vi "calculate_resistance.vi"(0 "Bare Resistance (MOhm)":dbl, 1 "Live Resistance":dbl, 2 "Solution Conductance \nS/m":dbl, 3 "Sealed Resistance (MOhm)":dbl, 5 "Membrane Thickness (nm)":dbl, 6 "Override":bool, 7 "Desired Pore Size (nm)":dbl) -> (4 "Boolean":bool, 10 "Capillary Diameter (nm)":dbl, 16 "Target Golovochenko  (MOhm)":dbl)   [LabVIEW 2016]
panel:
  out "Alpha":dbl
  out "Beta":dbl
  out "Membrane Thickness (m)":dbl
  out "Target Pore Diameter (m)":dbl
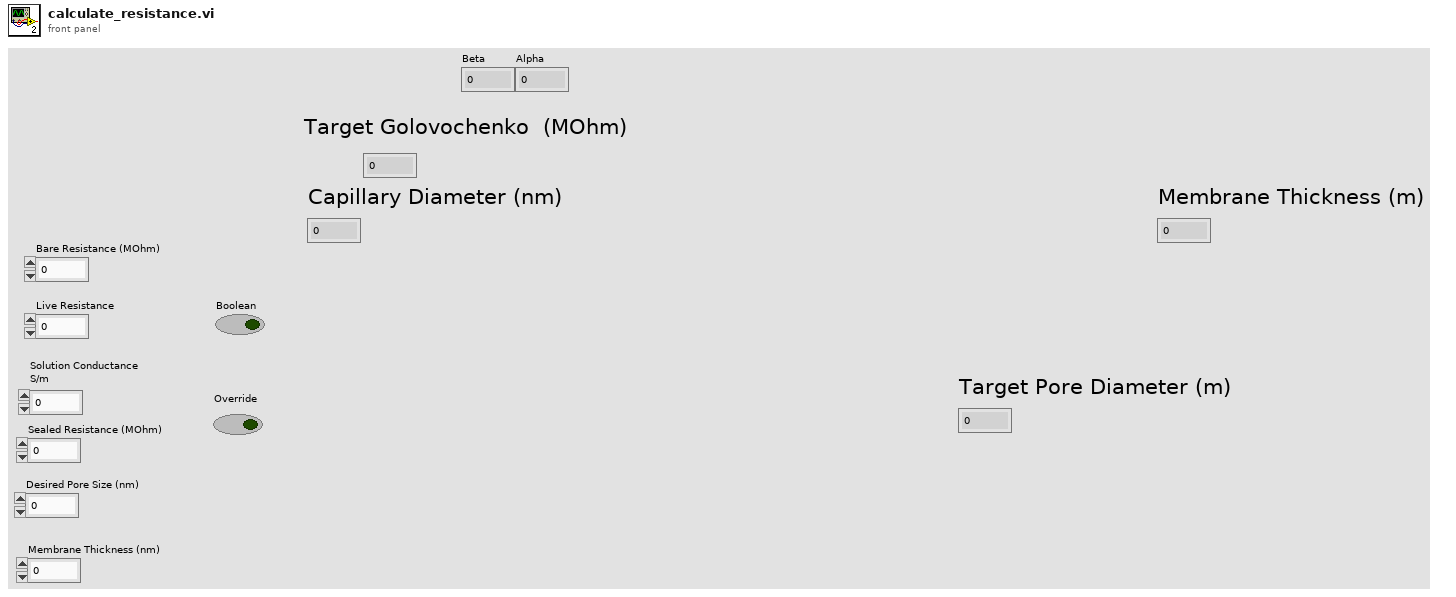
[diagram p1: front panel]
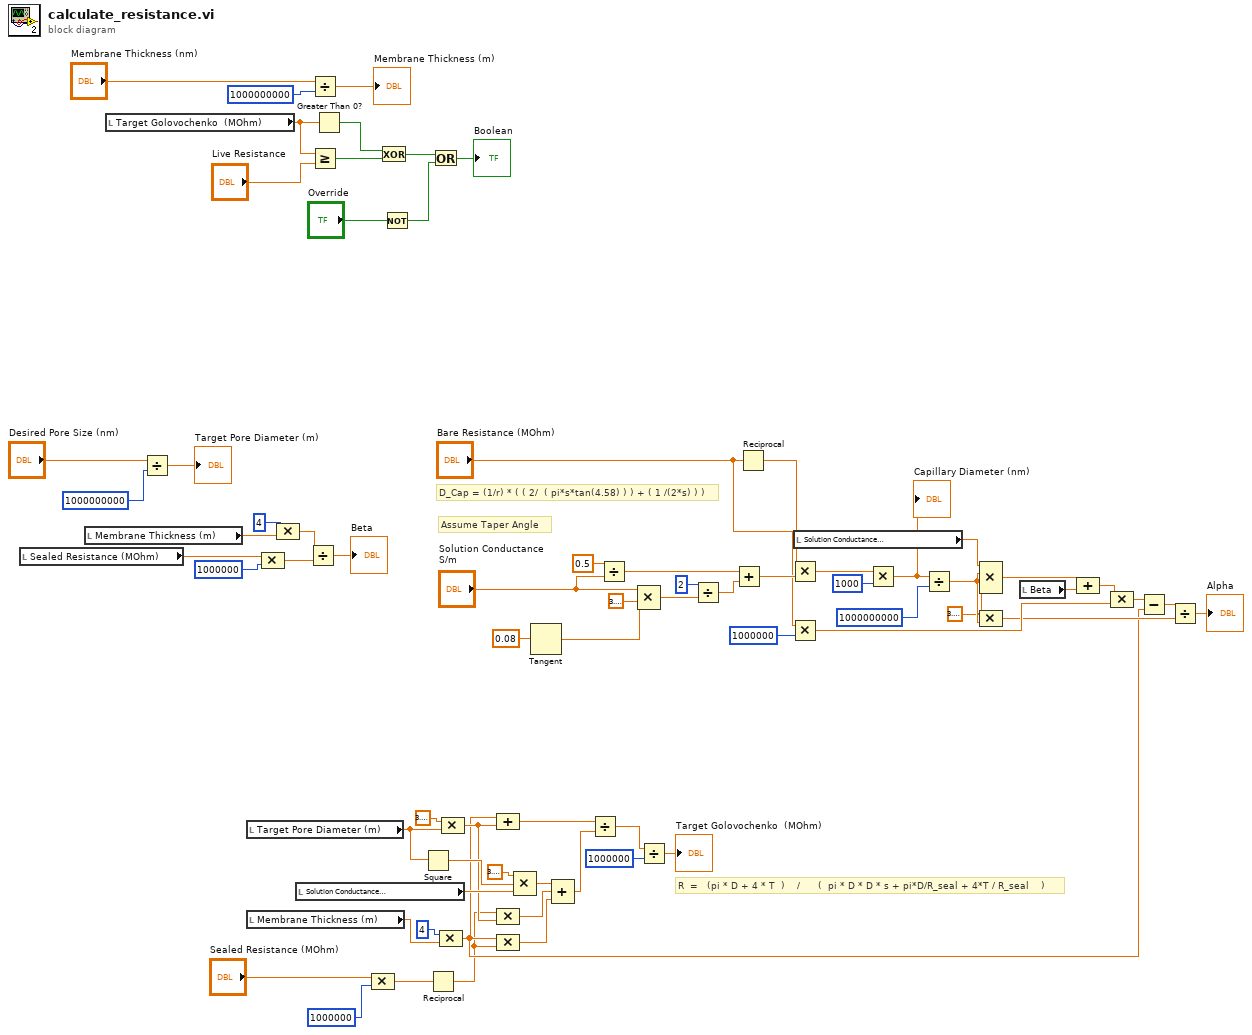
[diagram p0: block diagram]
diagram:
  w13 = 3.141592653589793
  # "D_Cap = (1/r) * ( ( 2/  ( pi*s*tan(4.58) ) ) + ( 1 /(2*s) ) )"
  # "R  =   (pi * D + 4 * T  )    /      (  pi * D * D * s + pi*D/R_seal + 4*T / R_seal    )"
  # "Assume Taper Angle"
  n1 = local read "Sealed Resistance (MOhm)"() -> (w48:dbl)
  n2 = local read "Membrane Thickness (m)"() -> (w29:dbl)
  n3 = local read "Target Golovochenko  (MOhm)"() -> (w58:dbl)
  n4 = Divide(x="Desired Pore Size (nm)", y=1000000000) -> (x/y=→"Target Pore Diameter (m)":dbl)
  n5 = local read "Target Pore Diameter (m)"() -> (w45:dbl)
  n6 = local read "Membrane Thickness (m)"() -> (w53:dbl)
  n7 = Compound Arithmetic op=MULTIPLY(w48, 1000000) -> (w27:dbl)
  n8 = Compound Arithmetic op=MULTIPLY(4, w29) -> (w28:dbl)
  n9 = local read "Solution Conductance \nS/m"() -> (w49:dbl)
  n10 = Divide(x=w28, y=w27) -> (x/y=→"Beta":dbl)
  n11 = Divide(x="Membrane Thickness (nm)", y=1000000000) -> (x/y=→"Membrane Thickness (m)":dbl)
  n12 = Greater Or Equal?(x=w58, y="Live Resistance") -> (x >= y?=w70:bool)
  n13 = Greater Than 0?(x=w58) -> (x > 0?=w69:bool)
  n14 = Compound Arithmetic op=MULTIPLY("Sealed Resistance (MOhm)", 1000000) -> (w7:dbl)
  n15 = Exclusive Or(1:w70, 2:w69) -> (0:w66:bool)
  n16 = Not(x="Override") -> (.not. x?=w65:bool)
  n17 = Square(x=w45) -> (x^2=w50:dbl)
  n18 = Reciprocal(x=w7) -> (1/x=w3:dbl)
  n19 = Or(x=w66, y=w65) -> (x .or. y?=→"Boolean":bool)
  n20 = Compound Arithmetic op=MULTIPLY(4, w53) -> (w4:dbl)
  n21 = Compound Arithmetic op=MULTIPLY(3.141592653589793, w45) -> (w6:dbl)
  n22 = Compound Arithmetic op=ADD(w4, w6) -> (w56:dbl)
  n23 = Compound Arithmetic op=MULTIPLY(w3, w6) -> (w5:dbl)
  n24 = Compound Arithmetic op=MULTIPLY(w4, w3) -> (w2:dbl)
  n25 = Compound Arithmetic op=MULTIPLY(3.141592653589793, w50, w49) -> (w10:dbl)
  n26 = Tangent(1:0.08) -> (0:w41:dbl)
  n27 = Compound Arithmetic op=ADD(w10, w5, w2) -> (w1:dbl)
  n28 = Divide(x=w56, y=w1) -> (x/y=w55:dbl)
  n29 = Divide(x=0.5, y="Solution Conductance \nS/m") -> (x/y=w37:dbl)
  n30 = Compound Arithmetic op=MULTIPLY("Solution Conductance \nS/m", 3.141592653589793, w41) -> (w39:dbl)
  n31 = Divide(x=w55, y=1000000) -> (x/y=→"Target Golovochenko  (MOhm)":dbl)
  n32 = Divide(x=2, y=w39) -> (x/y=w35:dbl)
  n33 = Add(x=w37, y=w35) -> (x+y=w34:dbl)
  n34 = Reciprocal(x="Bare Resistance (MOhm)") -> (1/x=w33:dbl)
  n35 = Multiply(x=w33, y=w34) -> (x*y=w32:dbl)
  n36 = Multiply(x="Bare Resistance (MOhm)", y=1000000) -> (x*y=w17:dbl)
  n37 = local read "Solution Conductance \nS/m"() -> (w21:dbl)
  n38 = Multiply(x=w32, y=1000) -> (x*y=w22:dbl)
  "Capillary Diameter (nm)" <- w22
  n39 = Divide(x=w22, y=1000000000) -> (x/y=w14:dbl)
  n40 = Compound Arithmetic op=MULTIPLY(w21, w14, w14, w13) -> (w20:dbl)
  n41 = Compound Arithmetic op=MULTIPLY(w13, w14) -> (w12:dbl)
  n42 = local read "Beta"() -> (w19:dbl)
  n43 = Compound Arithmetic op=ADD(w20, w19) -> (w18:dbl)
  n44 = Compound Arithmetic op=MULTIPLY(w18, w17) -> (w16:dbl)
  n45 = Subtract(x=w16, y=w4) -> (x-y=w15:dbl)
  n46 = Divide(x=w15, y=w12) -> (x/y=→"Alpha":dbl)
